vi "Periodic Tasks.vi"(8 "error in":errorcluster) -> ()   [LabVIEW 2018]
doc: "This VI runs in parallel to other tasks. It can contain as many user-defined periodic loops as you need. These can carry out PID or other sorts of timed response."
uses:
  PWF_Venom_LabVIEW/Public/TypeDefs/PwF_Venom_PIDParams.ctl
  DriveVenomDevRefs.ctl
  <vilib>/Rock Robotics/WPI/MotorControl/WPI_MotorControlDeviceRef.ctl
  <vilib>/Rock Robotics/WPI/MotorControl/WPI_MotorControlType.ctl
  <vilib>/Rock Robotics/SystemInterfaces/DIO/FPGA_DIOPWMChannel.ctl
  <vilib>/Rock Robotics/WPI/PWM/WPI_PWMDeadband.ctl
  <vilib>/Rock Robotics/SystemInterfaces/DIO/FPGA_DIOChannel.ctl
  DriveState.ctl
  PWF_Venom_LabVIEW/Public/TypeDefs/PwF_Venom_ControlMode.ctl
  88a8256b-dd6c-4d38-b021-9946be483166.vi
  72a4271e-8a2f-4e63-bef0-ab0047b3c302.vi
  4419bb08-cace-4eec-81e3-431b0f19f77f.vi
  43bb15c8-37b4-49b3-9761-3a694f89d06e.vi
  681b6e5e-4677-4682-a16d-7f94549bf0f7.vi
  f8245736-c666-4745-b76e-80ca56998d75.vi
  eff852b5-78a3-4797-aee6-6215f14f6dac.vi
  <vilib>/Array/Sort 2D Array - Pop Stack.vi
  <vilib>/Array/Sort 2D Array - Push Stack.vi
  <vilib>/Rock Robotics/WPI/Utilities/WPI_GetSetVariantRefNum.vi
  <vilib>/Rock Robotics/Network Tables/NT Read Numeric Array.vi
  <vilib>/Rock Robotics/WPI/ThirdParty/Phoenix-LabVIEW/Pigeon IMU/CTRE_PigeonIMU_GetFusedHeading.vi
  PWF_Venom_LabVIEW/PwF_Venom.lvlib
panel:
  in  "Set Angle":dbl(slide) scale=-180.0..180.0
  out "Degrees Off":dbl
  out "Center":dbl
  out "Height":dbl
  in  "Offset":dbl=182.0
  out "Waveform Chart":dbl(graph)=-0.0
  in  "PID Params":T1={"kP"=0.5, "kI"=0.0, "kD"=0.0, "kF"=0.184, "b"=0.0}
  in  "Track Width":dbl=2.3125
  in  "Tuning":dbl=10.0
  in  "Min Turn Radius":dbl=1.0
  in  "Max Wheel Velocity":dbl=4.0
  out "Avg Left Encoder (ft/s)":dbl
  out "Left Encoder (ft/s)":dbl
  in  "MinPower":dbl=0.063 format="%#_13g"
  out "dTime":u32=31
  out "Speed":dbl
  out "Position":dbl=-0.008333333333333333
  out "RightEncoderInches":dbl=0.005423177083333334
  out "LeftEncoderInches":dbl=0.037962239583333335
  out "RightEncoderRaw":dbl=0.25
  out "LeftEncoderRaw":dbl=1.75
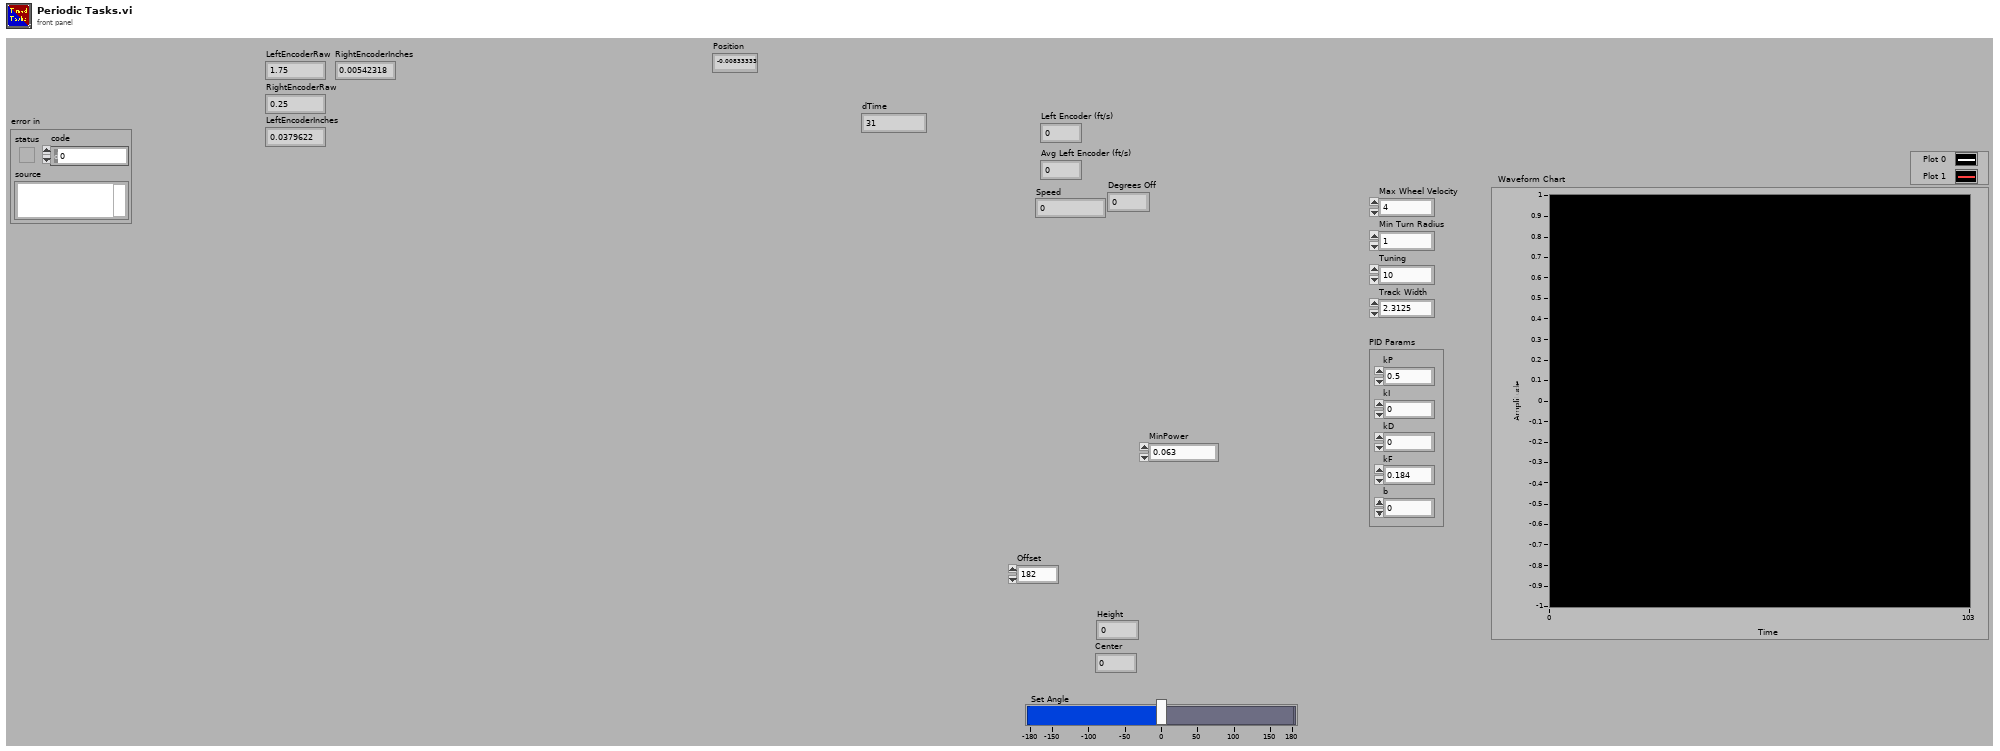
[diagram p1: front panel]
types:
  T1 = typedef "PwF_Venom.lvlib/PwF_Venom_PIDParams.ctl" = cluster{"kP":dbl, "kI":dbl, "kD":dbl, "kF":dbl, "b":dbl}
  T2 = cluster{"millisecond timer value":u32, "Distance":dbl}
  T3 = typedef "DriveVenomDevRefs.ctl" = cluster{"FrontLeft":T4, "FrontRight":T4}
  T4 = typedef "WPI_MotorControlDeviceRef.ctl" = cluster{"DeviceStatus":errorcluster, "Type":T5, "PWM":cluster{"PWM Channel":T6, "DeadBand":T7}, "CAN":cluster{"Device Number":u8, "SetOutput VI Ref":variant, "GetOutput VI Ref":variant, "Enable VI Ref":variant, "Disable VI Ref":variant, "Data":variant}, "Invert":bool, "DIO PWM":cluster{"PWM \"Enable\" Channel":T6, "DIOChannel":T8, "PWM Rate":dbl}}
  T5 = typedef "WPI_MotorControlType.ctl" = enum16{"PWM", "CAN", "DIO PWM"}
  T6 = typedef "FPGA_DIOPWMChannel.ctl" = enum8{"PWM 0", "PWM 1", "PWM 2", "PWM 3", "PWM 4", "PWM 5", "PWM 6", "PWM 7", "PWM 8", "PWM 9", "PWM MXP 0", "PWM MXP 1", "PWM MXP 2", "PWM MXP 3", "PWM MXP 4", "PWM MXP 5", "PWM MXP 6", "PWM MXP 7", "PWM MXP 8", "PWM MXP 9", "Invalid"}
  T7 = typedef "WPI_PWMDeadband.ctl" = cluster{"Name":string, "maxPositivePwm":i32, "minPositivePwm":i32, "centerPwm":i32, "maxNegativePwm":i32, "minNegativePwm":i32, "angularRange":u16}
  T8 = typedef "FPGA_DIOChannel.ctl" = enum8{"DIO 0", "DIO 1", "DIO 2", "DIO 3", "DIO 4", "DIO 5", "DIO 6", "DIO 7", "DIO 8", "DIO 9", "DIO MXP 0", "DIO MXP 1", "DIO MXP 2", "DIO MXP 3", "DIO MXP 4", "DIO MXP 5", "DIO MXP 6", "DIO MXP 7", "DIO MXP 8", "DIO MXP 9", "DIO MXP 10", "DIO MXP 11", "DIO MXP 12", "DIO MXP 13", "DIO MXP 14", "DIO MXP 15", "SPI Port CS1", "SPI Port CS2", "SPI Port CS3", "SPI Port MISO", "SPI Port MOSI", "Invalid"}
  T9 = typedef "WPI_I2CDevRef.ctl" = cluster{"DevStatus":errorcluster, "Device Address":u8, "Handle":i32, "I2C Bus":T10}
  T10 = typedef "i2c_bus.ctl" = enum16{"I2C On-Board", "I2C MXP", "Invalid"}
  T11 = typedef "CTRE_PigeonIMU_DeviceRef.ctl" = cluster{"DeviceStatus":errorcluster, "Device Number":u8, "Type":T12, "Device ID":u32, "Handle":u64, "UsageFrame":u32, "Library Path":path}
  T12 = typedef "CTRE_PigeonIMU_ConnectionType.ctl" = u32
  T13 = typedef "WPI_EncoderDevRef.ctl" = cluster{"DevStatus":errorcluster, "EncoderIndex":T14, "CounterIndex":T15, "DistancePerCount":dbl, "Decoding Type":T16}
  T14 = typedef "FPGA_EncoderIdx.ctl" = enum8{"Enc 0", "Enc 1", "Enc 2", "Enc 3", "Enc 4", "Enc 5", "Enc 6", "Enc 7", "Invalid"}
  T15 = typedef "FPGA_CounterCtrSystemIndex.ctl" = enum8{"Ctr 0", "Ctr 1", "Ctr 2", "Ctr 3", "Ctr 4", "Ctr 5", "Ctr 6", "Ctr 7", "Invalid"}
  T16 = typedef "WPI_EncoderType.ctl" = enum16{"1x", "2x", "4x"}
  T17 = typedef "WPI_JoystickDevRef.ctl" = cluster{"Device":T18}
  T18 = typedef "WPI_JoystickDeviceEnum.ctl" = enum16{"USB 0", "USB 1", "USB 2", "USB 3", "USB 4", "USB 5"}
  T19 = cluster{"millisecond timer value":u32, "Distance":dbl}[]
  T20 = enum16{"[0, 360]", "[-180, 180]", "[0, 2PI]", "[-PI, PI]"}
  T21 = cluster{"Heading":dbl, "Valid?":bool, "Fusing?":bool}
  T22 = typedef "DriveState.ctl" = enum16{"Manual", "Velocity", "Test Static Friction", "Do Nothing"}
  T23 = typedef "PwF_Venom.lvlib/PwF_Venom_ControlMode.ctl" = u8
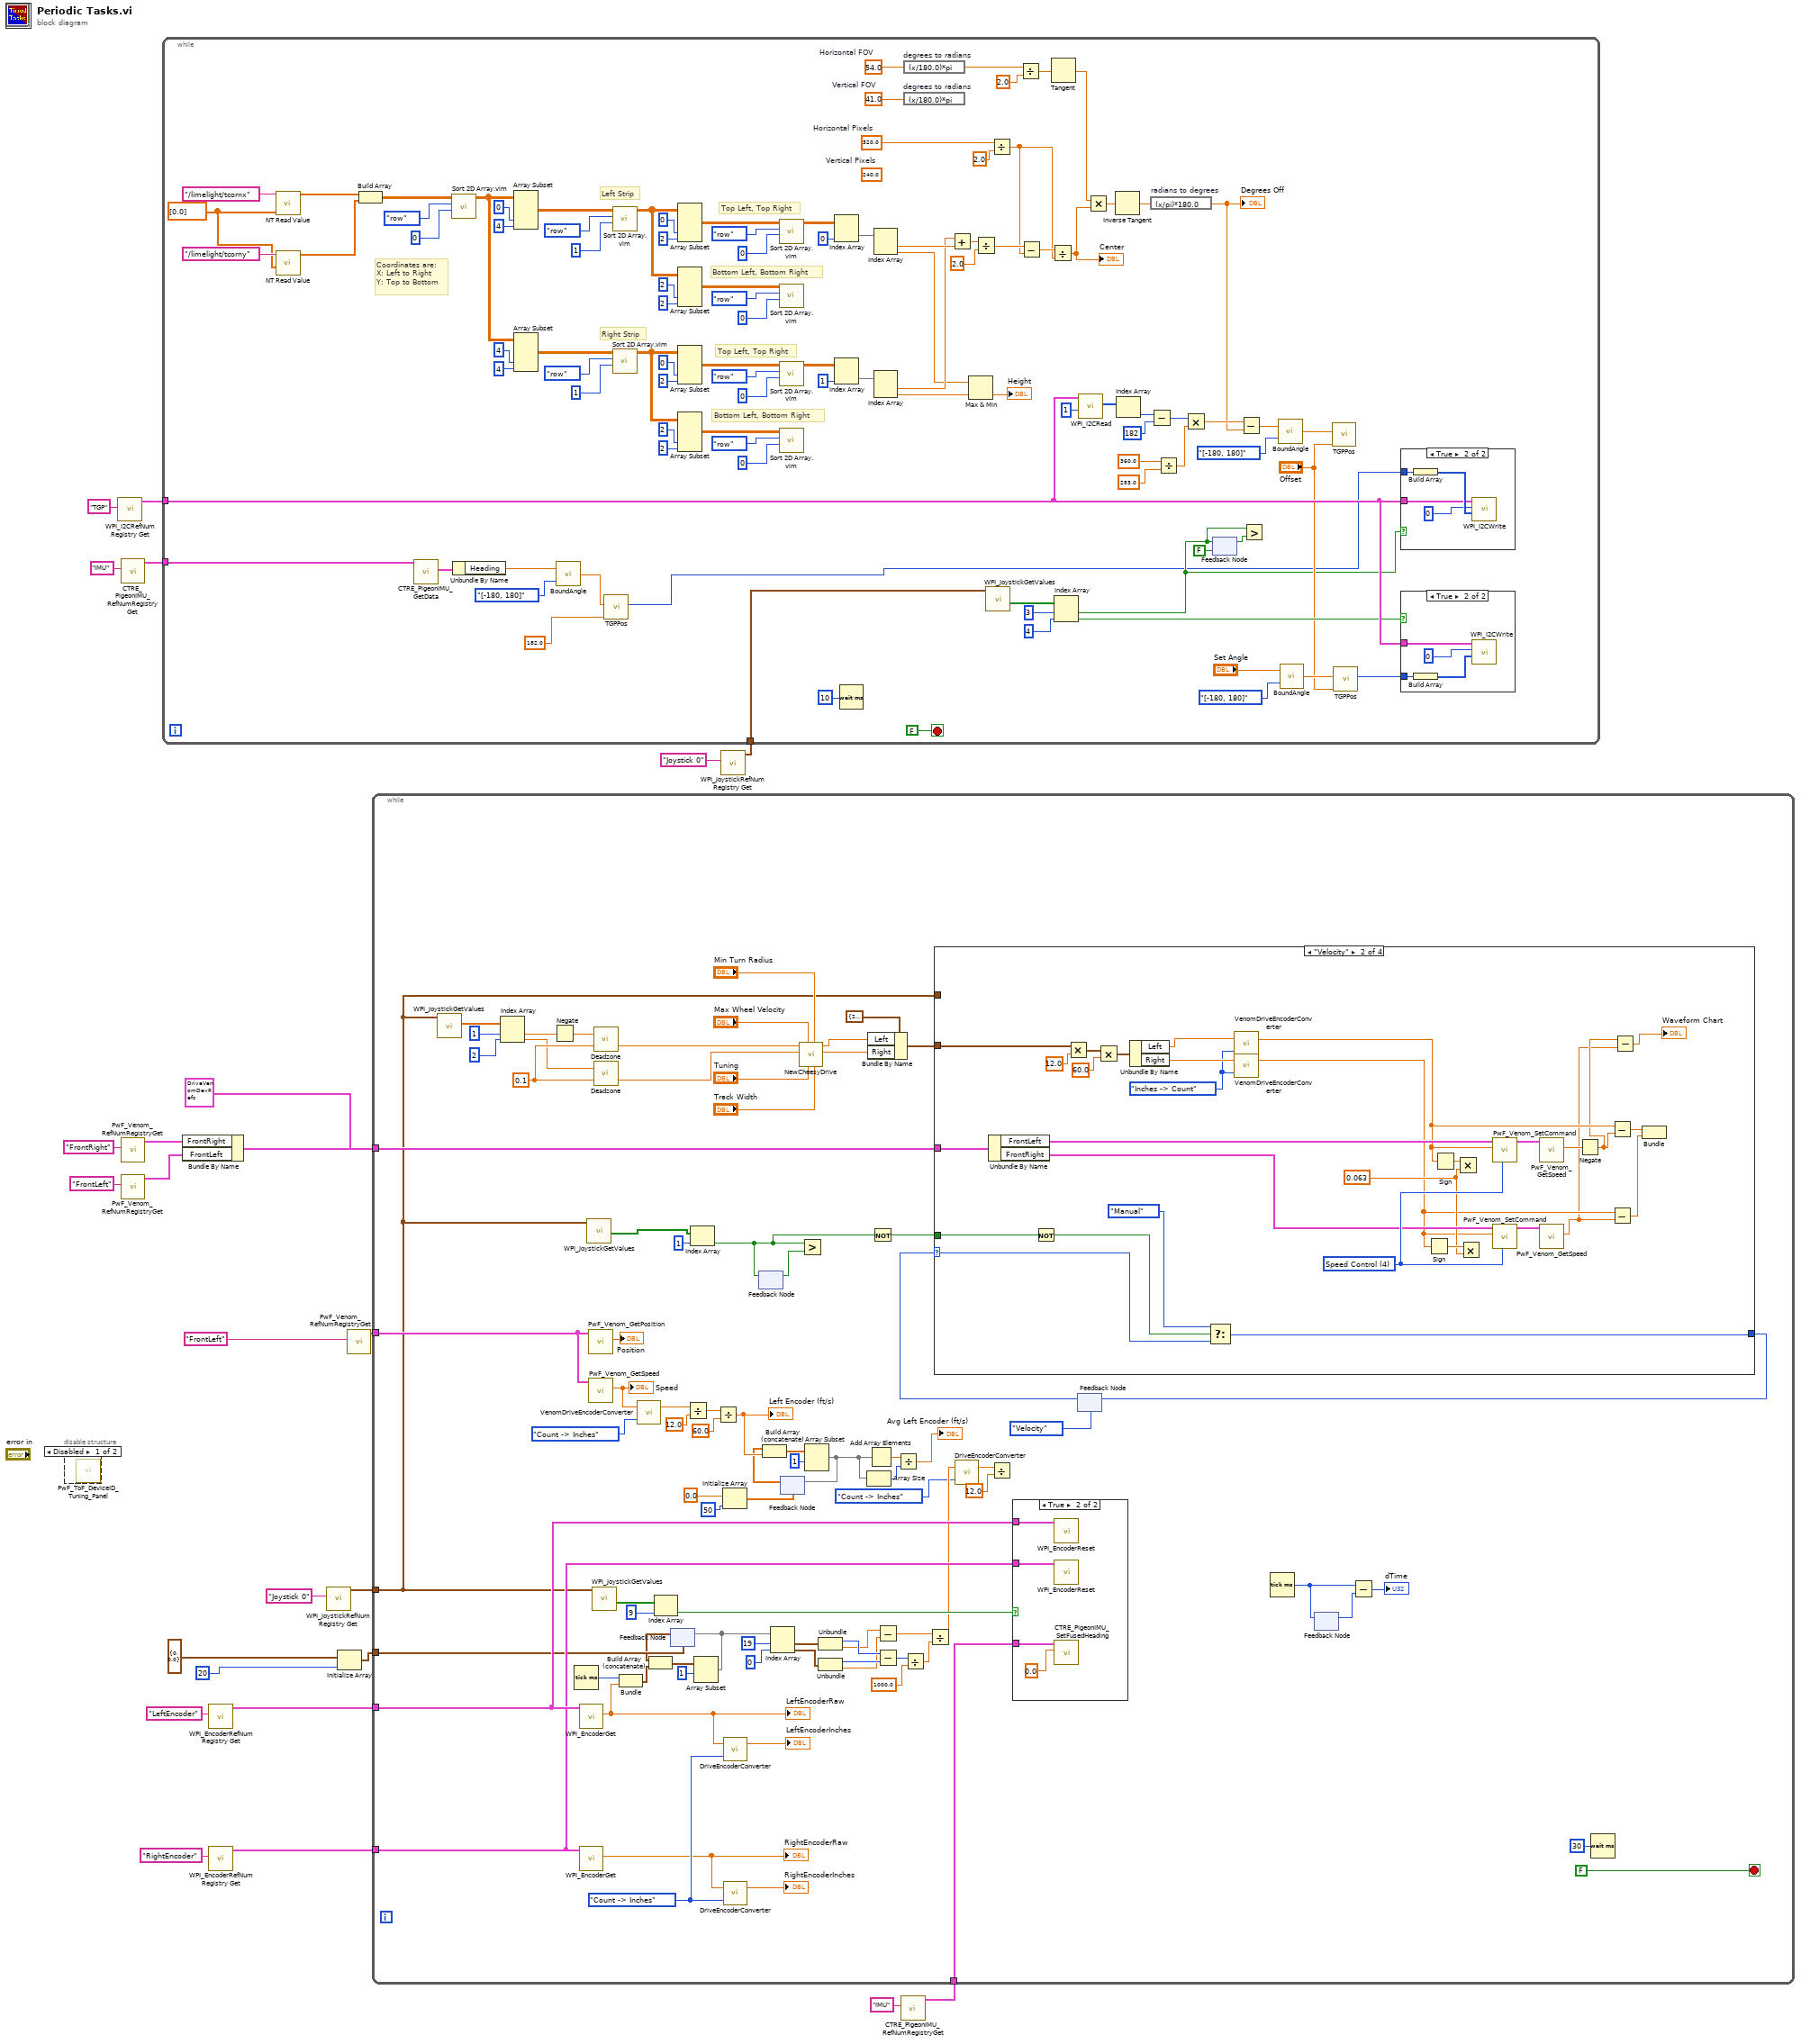
[diagram p0: block diagram]
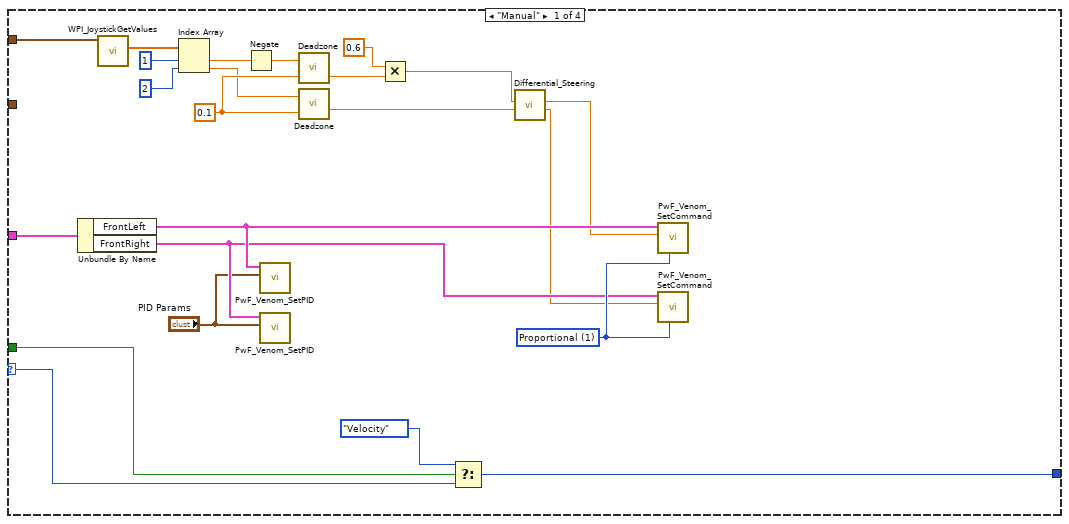
[diagram p6: hidden frame]
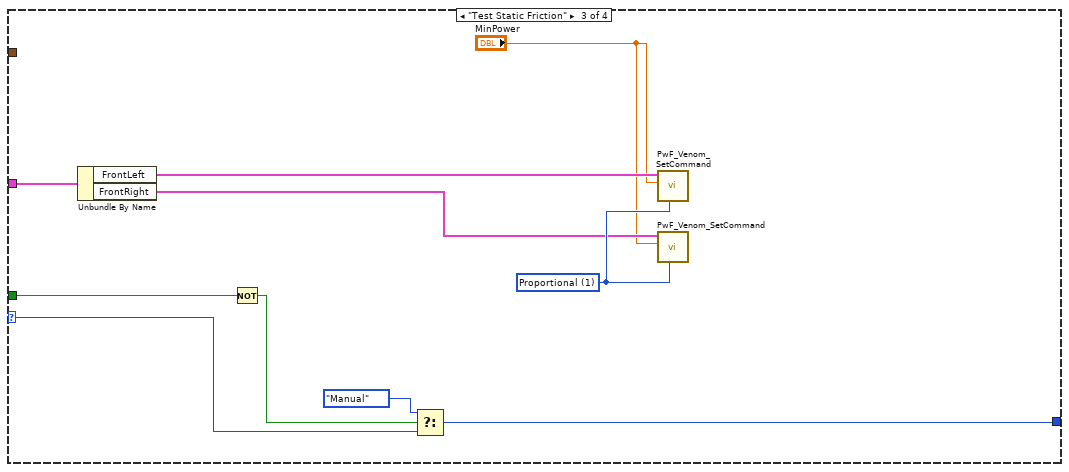
[diagram p7: hidden frame]
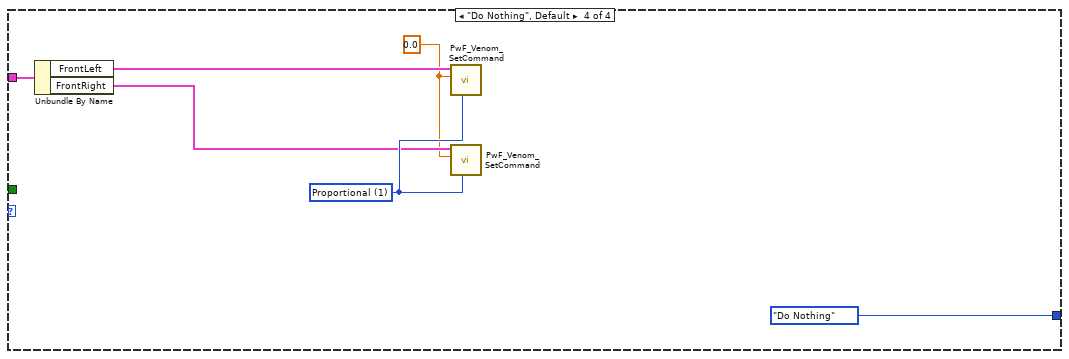
[diagram p8: hidden frame]
diagram:
  n1 = disable-structure shown="Disabled" {
    frame Disabled {
      n2 = call "PwF_ToF_DeviceID_Tuning_Panel.vi"() -> ()  [unwired: 12 in]
    }
    frame Enabled {
    }
  }
  n3 = call <vilib>:"WPI_I2CRefNum Registry Get.vi"("refnum name"="TGP") -> ("I2CDevRef"=w4:T9)  [unwired: 9 in, 1 out]
  n4 = call <vilib>:"CTRE_PigeonIMU_RefNumRegistryGet.vi"("refnum name"="IMU") -> ("PigeonIMUDevRef"=w3:T11)  [unwired: 9 in, 1 out]
  n5 = call "PwF_Venom_RefNumRegistryGet.vi"("refnum name"="FrontRight") -> ("PwFVenomDevRefOut"=w12:T4)  [unwired: 9 in, 1 out]
  n6 = call "PwF_Venom_RefNumRegistryGet.vi"("refnum name"="FrontLeft") -> ("PwFVenomDevRefOut"=w11:T4)  [unwired: 9 in, 1 out]
  n7 = Bundle By Name(cluster=T3 {"FrontLeft"={"DeviceStatus"={"status"=FALSE, "code"=0, "source"=""}, "Type"=enum."PWM", "PWM"={"PWM Channel"=enum."Invalid", "DeadBand"={"Name"="", "maxPositivePwm"=0, "minPositivePwm"=0, "centerPwm"=0, "maxNegativePwm"=0, "minNegativePwm"=0, "angularRange"=0}}, "CAN"={"Device Number"=0, "SetOutput VI Ref"=variant(refnum<vi> refnum), "GetOutput VI Ref"=variant(refnum<vi> refnum), "Enable VI Ref"=variant(refnum<vi> refnum), "Disable VI Ref"=variant(refnum<vi> refnum), "Data"=variant}, "Invert"=FALSE, "DIO PWM"={"PWM \"Enable\" Channel"=enum."Invalid", "DIOChannel"=enum."Invalid", "PWM Rate"=0.0}}, "FrontRight"={"DeviceStatus"={"status"=FALSE, "code"=0, "source"=""}, "Type"=enum."PWM", "PWM"={"PWM Channel"=enum."Invalid", "DeadBand"={"Name"="", "maxPositivePwm"=0, "minPositivePwm"=0, "centerPwm"=0, "maxNegativePwm"=0, "minNegativePwm"=0, "angularRange"=0}}, "CAN"={"Device Number"=0, "SetOutput VI Ref"=variant(refnum<vi> refnum), "GetOutput VI Ref"=variant(refnum<vi> refnum), "Enable VI Ref"=variant(refnum<vi> refnum), "Disable VI Ref"=variant(refnum<vi> refnum), "Data"=variant}, "Invert"=FALSE, "DIO PWM"={"PWM \"Enable\" Channel"=enum."Invalid", "DIOChannel"=enum."Invalid", "PWM Rate"=0.0}}} ("DriveVenomDevRefs"), "FrontRight"=w12, "FrontLeft"=w11) -> (w10:T3)
  n8 = call <vilib>:"WPI_EncoderRefNum Registry Get.vi"("refnum name"="LeftEncoder") -> ("EncoderDevRef"=w24:T13)  [unwired: 9 in, 1 out]
  n9 = call <vilib>:"WPI_EncoderRefNum Registry Get.vi"("refnum name"="RightEncoder") -> ("EncoderDevRef"=w23:T13)  [unwired: 9 in, 1 out]
  n10 = call <vilib>:"WPI_JoystickRefNum Registry Get.vi"("refnum name"="Joystick 0") -> ("JoystickDevRef"=w18:T17)  [unwired: 9 in, 1 out]
  n11 = Initialize Array(T2 {"millisecond timer value"=0, "Distance"=0.0}, 20 ("dimension size")) -> (w7:T19)
  n12 = call "PwF_Venom_RefNumRegistryGet.vi"("refnum name"="FrontLeft") -> ("PwFVenomDevRefOut"=w17:T4)  [unwired: 9 in, 1 out]
  n13 = call <vilib>:"WPI_JoystickRefNum Registry Get.vi"("refnum name"="Joystick 0") -> ("JoystickDevRef"=w1:T17)  [unwired: 9 in, 1 out]
  n14 = while {
    tunnel: w4 -> [w46]
    tunnel: w3 -> [w123]
    tunnel: w1 -> [w35]
    stop <- FALSE stop-if-true
    (unwired) 240.0  # Vertical Pixels
    w58 = 320.0  # Horizontal Pixels
    w67 = 41.0  # Vertical FOV
    w70 = 54.0  # Horizontal FOV
    w118 = dbl[] [0.0] ("Default Value")
    # "Coordinates are:\nX: Left to Right\nY: Top to Bottom"
    # "Top Left, Top Right"
    # "Bottom Left, Bottom Right"
    # "Top Left, Top Right"
    # "Bottom Left, Bottom Right"
    # "Right Strip"
    # "Left Strip"
    n15 = call-poly <vilib>:"NT Read Value.vi"("Default Value"=w118, "Name"="/limelight/tcornx") -> ("Numeric Array"=w120:dbl[])  [unwired: 8 in, 1 out]
    n16 = call-poly <vilib>:"NT Read Value.vi"("Default Value"=w118, "Name"="/limelight/tcorny") -> ("Numeric Array"=w119:dbl[])  [unwired: 8 in, 1 out]
    n17 = Build Array(w120, w119) -> (w115:dbl[][])
    n18 = call-poly <vilib>:"CTRE_PigeonIMU_GetData.vi"("PigeonIMUDevRef"=w123) -> ("Fused Heading"=w125:T21)  [unwired: 8 in, 2 out]
    n19 = call "Sort 2D Array.vim"("index"=0, "dimension to index (column)"=enum16{"column", "row"}."row", "2D array"=w115) -> ("sorted 2D array"=w110:dbl[][])  [unwired: 7 in, 1 out]
    n20 = Unbundle By Name(w125) -> ("Heading"=w126:dbl)
    n21 = Array Subset(array=w110, index (col)=0 ("index"), length (col)=4 ("index")) -> (w107:dbl[][])  [unwired: 2 in]
    n22 = Array Subset(array=w110, index (col)=4 ("index"), length (col)=4 ("index")) -> (w104:dbl[][])  [unwired: 2 in]
    n23 = call <userlib>:"BoundAngle.vi"("Type"=T20."[-180, 180]", "Angle"=w126) -> ("Bound Angle"=w28:dbl)
    n24 = call "TGPPos.vi"("Offset"=182.0 ("Offset 2"), "Angle (-179 - 180)"=w28) -> ("TGP Pos"=w27:u8)  [unwired: 9 in]
    n25 = call "Sort 2D Array.vim"("index"=1, "dimension to index (column)"=enum16{"column", "row"}."row", "2D array"=w107) -> ("sorted 2D array"=w99:dbl[][])  [unwired: 7 in, 1 out]
    n26 = call "Sort 2D Array.vim"("index"=1, "dimension to index (column)"=enum16{"column", "row"}."row", "2D array"=w104) -> ("sorted 2D array"=w94:dbl[][])  [unwired: 7 in, 1 out]
    n27 = Array Subset(array=w99, index (col)=0 ("index"), length (col)=2 ("index")) -> (w91:dbl[][])  [unwired: 2 in]
    n28 = Array Subset(array=w99, index (col)=2 ("index"), length (col)=2 ("index")) -> (w88:dbl[][])  [unwired: 2 in]
    n29 = Array Subset(array=w94, index (col)=0 ("index"), length (col)=2 ("index")) -> (w83:dbl[][])  [unwired: 2 in]
    n30 = Array Subset(array=w94, index (col)=2 ("index"), length (col)=2 ("index")) -> (w82:dbl[][])  [unwired: 2 in]
    n31 = call "Sort 2D Array.vim"("index"=0, "dimension to index (column)"=enum16{"column", "row"}."row", "2D array"=w91) -> ("sorted 2D array"=w79:dbl[][])  [unwired: 7 in, 1 out]
    n32 = call "Sort 2D Array.vim"("index"=0, "dimension to index (column)"=enum16{"column", "row"}."row", "2D array"=w88) -> ()  [unwired: 7 in, 2 out]
    n33 = call "Sort 2D Array.vim"("index"=0, "dimension to index (column)"=enum16{"column", "row"}."row", "2D array"=w83) -> ("sorted 2D array"=w78:dbl[][])  [unwired: 7 in, 1 out]
    n34 = call "Sort 2D Array.vim"("index"=0, "dimension to index (column)"=enum16{"column", "row"}."row", "2D array"=w82) -> ()  [unwired: 7 in, 2 out]
    n35 = Index Array(array=w79, index (col)=0 ("disabled index (col)")) -> (element=w77:dbl[])  [unwired: 1 in]
    n36 = Index Array(array=w78, index (col)=1 ("disabled index (col)")) -> (element=w76:dbl[])  [unwired: 1 in]
    n37 = Wait (ms)(milliseconds to wait=u32 10) -> ()  [unwired: 1 out]
    n38 = Index Array(array=w77) -> (element #1=w75:dbl, element #2=w73:dbl)  [unwired: 2 in]
    n39 = Index Array(array=w76) -> (element #1=w74:dbl, element #2=w72:dbl)  [unwired: 2 in]
    n40 = expression code="(x/180.0)*pi" "degrees to radians"(w70) -> (w68:dbl)
    n41 = expression code="(x/180.0)*pi" "degrees to radians"(w67) -> ()  [unwired: 1 out]
    n42 = Add(x=w74, y=w75) -> (x+y=w62:dbl)
    n43 = Max & Min(x=w73, y=w72) -> (min(x,y)=→"Height":dbl)  [unwired: 1 out]
    n44 = Divide(x=w62, y=2.0 ("x+y")) -> (x/y=w60:dbl)
    n45 = call <vilib>:"WPI_JoystickGetValues.vi"("JoystickDevRef"=w35) -> ("Buttons"=w40:bool[])  [unwired: 6 in, 4 out]
    n46 = Divide(x=w58, y=2.0) -> (x/y=w55:dbl)
    n47 = Divide(x=w68, y=2.0) -> (x/y=w66:dbl)
    n48 = Subtract(x=w60, y=w55) -> (x-y=w59:dbl)
    n49 = Divide(x=w59, y=w55) -> (x/y=w56:dbl)
    "Center" <- w56
    n50 = Tangent(1:w66) -> (0:w65:dbl)
    n51 = Index Array(array=w40, index #1=3 ("index"), index #2=4 ("index")) -> (element #1=w29:bool, element #2=w36:bool)
    n52 = call <vilib>:"WPI_I2CRead.vi"("I2CBytesToRead"=u8 1, "I2CDevRef"=w46) -> ("Data Out"=w54:u8[])  [unwired: 7 in, 2 out]
    n53 = Multiply(x=w65, y=w56) -> (x*y=w64:dbl)
    n54 = Inverse Tangent(1:w64) -> (0:w63:dbl)
    n55 = Index Array(array=w54) -> (element=w51:u8)  [unwired: 1 in]
    n56 = Subtract(x=w51, y=u8 182) -> (x-y=w32:u8)
    n57 = expression code="(x/pi)*180.0" "radians to degrees"(w63) -> (w33:dbl)
    "Degrees Off" <- w33
    n58 = Divide(x=360.0, y=253.0 ("x")) -> (x/y=w50:dbl)
    n59 = Multiply(x=w32, y=w50) -> (x*y=w34:dbl)
    n60 = feedback-in #1(w29) -> ()
    n61 = feedback #1(FALSE) -> (w38:bool)
    n62 = Subtract(x=w34, y=w33) -> (x-y=w48:dbl)
    n63 = Greater?(x=w29, y=w38) -> ()  [unwired: 1 out]
    n64 = call <userlib>:"BoundAngle.vi"("Type"=T20."[-180, 180]", "Angle"=w48) -> ("Bound Angle"=w47:dbl)
    n65 = call <userlib>:"BoundAngle.vi"("Type"=T20."[-180, 180]", "Angle"="Set Angle") -> ("Bound Angle"=w44:dbl)
    n66 = call "TGPPos.vi"("Offset"="Offset", "Angle (-179 - 180)"=w47) -> ()  [unwired: 9 in, 1 out]
    n67 = call "TGPPos.vi"("Offset"="Offset", "Angle (-179 - 180)"=w44) -> ("TGP Pos"=w42:u8)  [unwired: 9 in]
    n68 = case shown="True" w29 {
      tunnel: w46 -> [_ w135]
      tunnel: w27 -> [_ w134]
      frame False {
      }
      frame True {
        n69 = Build Array(w134) -> (w137:u8[])
        n70 = call <vilib>:"WPI_I2CWrite.vi"("I2CDataToSend"=w137, "I2CRegister"=u8 0, "I2CDevRef"=w135) -> ()  [unwired: 7 in, 2 out]
      }
    }
    n71 = case shown="True" w36 {
      tunnel: w42 -> [_ w131]
      tunnel: w46 -> [_ w130]
      frame False {
      }
      frame True {
        n72 = Build Array(w131) -> (w133:u8[])
        n73 = call <vilib>:"WPI_I2CWrite.vi"("I2CDataToSend"=w133, "I2CRegister"=u8 0, "I2CDevRef"=w130) -> ()  [unwired: 7 in, 2 out]
      }
    }
  }
  n74 = call <vilib>:"CTRE_PigeonIMU_RefNumRegistryGet.vi"("refnum name"="IMU") -> ("PigeonIMUDevRef"=w20:T11)  [unwired: 9 in, 1 out]
  n75 = while {
    tunnel: w24 -> [w220]
    tunnel: w23 -> [w219]
    tunnel: w20 -> [w218]
    tunnel: w18 -> [w187]
    tunnel: w17 -> [w217]
    tunnel: w10 -> [w216]
    tunnel: w7 -> [w209]
    stop <- FALSE stop-if-true
    w186 = enum16{"Count -> Inches", "Inches -> Count"}."Count -> Inches" ("Mode")
    w196 = 0.1 ("Deadzone")
    n76 = call <vilib>:"WPI_JoystickGetValues.vi"("JoystickDevRef"=w187) -> ("Axes"=w197:dbl[])  [unwired: 6 in, 4 out]
    n77 = Index Array(array=w197, index #1=1 ("index"), index #2=2 ("index")) -> (element #1=w198:dbl, element #2=w192:dbl)
    n78 = Negate(x=w198) -> (-x=w193:dbl)
    n79 = Tick Count (ms)() -> (millisecond timer value=w172:u32)
    n80 = call <vilib>:"WPI_EncoderGet.vi"("EncoderDevRef"=w220) -> ("Distance"=w173:dbl)  [unwired: 5 in, 5 out]
    "LeftEncoderRaw" <- w173
    n81 = call <vilib>:"WPI_EncoderGet.vi"("EncoderDevRef"=w219) -> ("Distance"=w181:dbl)  [unwired: 5 in, 5 out]
    "RightEncoderRaw" <- w181
    n82 = call <vilib>:"WPI_JoystickGetValues.vi"("JoystickDevRef"=w187) -> ("Buttons"=w188:bool[])  [unwired: 6 in, 4 out]
    n83 = call "PwF_Venom_GetPosition.vi"("PwFVenomDevRefIn"=w217) -> ("Position"=→"Position":dbl)  [unwired: 8 in, 2 out]
    n84 = call "PwF_Venom_GetSpeed.vi"("PwFVenomDevRefIn"=w217) -> ("Speed"=w142:dbl)  [unwired: 8 in, 2 out]
    "Speed" <- w142
    n85 = call <vilib>:"WPI_JoystickGetValues.vi"("JoystickDevRef"=w187) -> ("Buttons"=w177:bool[])  [unwired: 6 in, 4 out]
    n86 = call <userlib>:"Deadzone.vi"("Deadzone"=w196, "Input Signal"=w193) -> ("Output Signal"=w191:dbl)  [unwired: 1 out]
    n87 = call <userlib>:"Deadzone.vi"("Deadzone"=w196, "Input Signal"=w192) -> ("Output Signal"=w190:dbl)  [unwired: 1 out]
    n88 = Bundle("millisecond timer value"=w172, "Distance"=w173) -> (w171:T2)  [unwired: 1 in]
    n89 = call "VenomDriveEncoderConverter.vi"("Mode"=enum16{"Count -> Inches", "Inches -> Count"}."Count -> Inches", "Input"=w142) -> ("Output"=w141:dbl)  [unwired: 1 in]
    n90 = Index Array(array=w177, index=9) -> (element=w182:bool)
    n91 = feedback #2(w209) -> (w174:T19)
    n92 = Build Array (concatenate)(w174, w171) -> (w176:T19)
    n93 = Divide(x=w141, y=12.0) -> (x/y=w139:dbl)
    n94 = Index Array(array=w188, index=1) -> (element=w210:bool)
    n95 = Array Subset(array=w176, index=1) -> (w170:T19)  [unwired: 1 in]
    n96 = feedback-in #2(w170) -> ()
    n97 = Divide(x=w139, y=60.0) -> (x/y=w208:dbl)
    "Left Encoder (ft/s)" <- w208
    n98 = Initialize Array(0.0 ("y"), 50 ("dimension size")) -> (w148:dbl[])
    n99 = call "DriveEncoderConverter.vi"("Mode"=w186, "Input"=w173) -> ("Output"=→"LeftEncoderInches":dbl)  [unwired: 1 in]
    n100 = call "DriveEncoderConverter.vi"("Mode"=w186, "Input"=w181) -> ("Output"=→"RightEncoderInches":dbl)  [unwired: 1 in]
    n101 = feedback-in #3(w210) -> ()
    n102 = feedback #3() -> (w211:bool)  [unwired: 1 in]
    n103 = Index Array(array=w170, index #1=19 ("index"), index #2=0 ("index")) -> (element #1=w167:T2, element #2=w166:T2)
    n104 = feedback #4(w148) -> (w151:dbl[])
    n105 = Build Array (concatenate)(w151, w208) -> (w153:dbl[])
    n106 = call "NewCheesyDrive.vi"("Track Width"="Track Width", "Min Turn Radius"="Min Turn Radius", "Tuning"="Tuning", "Max Wheel Velocity"="Max Wheel Velocity", "X"=w190, "Y"=w191) -> ("Right Speed"=w204:dbl, "Left Speed"=w203:dbl)  [unwired: 4 in]
    n107 = Greater?(x=w210, y=w211) -> ()  [unwired: 1 out]
    n108 = Array Subset(array=w153, index=1) -> (w147:dbl[])  [unwired: 1 in]
    n109 = feedback-in #4(w147) -> ()
    n110 = Unbundle(w167) -> ("millisecond timer value"=w165:u32, "Distance"=w163:dbl)
    n111 = Unbundle(w166) -> ("millisecond timer value"=w164:u32, "Distance"=w162:dbl)
    n112 = Array Size(array=w147) -> (size(s)=w145:i32)
    n113 = Bundle By Name(cluster=cluster{"Left":dbl, "Right":dbl} {"Left"=2.0, "Right"=2.0} ("input cluster"), "Left"=w203, "Right"=w204) -> (w205:cluster{"Left":dbl, "Right":dbl})
    n114 = Add Array Elements(numeric array=w147) -> (sum=w146:dbl)
    n115 = Not(x=w210) -> (.not. x?=w189:bool)
    n116 = Subtract(x=w163, y=w162) -> (x-y=w161:dbl)
    n117 = Subtract(x=w165, y=w164) -> (x-y=w156:u32)
    n118 = Divide(x=w146, y=w145) -> (x/y=→"Avg Left Encoder (ft/s)":dbl)
    n119 = Divide(x=w156, y=1000.0) -> (x/y=w155:dbl)
    n120 = Divide(x=w161, y=w155) -> (x/y=w160:dbl)
    n121 = call "DriveEncoderConverter.vi"("Mode"=enum16{"Count -> Inches", "Inches -> Count"}."Count -> Inches", "Input"=w160) -> ("Output"=w158:dbl)  [unwired: 1 in]
    n122 = Divide(x=w158, y=12.0) -> ()  [unwired: 1 out]
    n123 = case shown="True" w182 {
      tunnel: w220 -> [_ w226]
      tunnel: w219 -> [_ w225]
      tunnel: w218 -> [_ w224]
      frame False {
      }
      frame True {
        n124 = call <vilib>:"WPI_EncoderReset.vi"("EncoderDevRef"=w226) -> ()  [unwired: 9 in, 2 out]
        n125 = call <vilib>:"WPI_EncoderReset.vi"("EncoderDevRef"=w225) -> ()  [unwired: 9 in, 2 out]
        n126 = call <vilib>:"CTRE_PigeonIMU_SetFusedHeading.vi"("Value"=0.0, "PigeonIMUDevRef 2"=w224) -> ()  [unwired: 8 in, 2 out]
      }
    }
    n127 = feedback #5(DriveState."Velocity") -> (w214:T22)
    n128 = case shown="\"Velocity\"" w214 {
      selector: w214 -> [w235 w274 w283 _]
      tunnel: w187 -> [w243 _ _ _]
      tunnel: w216 -> [w242 w278 w288 w294]
      tunnel: w205 -> [_ w265 _ _]
      tunnel: [w237 w275 w284 DriveState."Do Nothing"] -> w213
      tunnel: w189 -> [w236 w273 w282 _]
      frame "Manual" {
        w247 = 0.1 ("Deadzone")
        w246 = T23 1 items=["Disabled"=0, "Proportional"=1, "Current Control"=3, "Speed Control"=4, "Position Control"=5, "Motion Profile"=6, "Follow The Leader"=7, "Voltage Control"=8] ("PwF Venom Control Mode")
        n129 = Unbundle By Name(w242) -> ("FrontLeft"=w233:T4, "FrontRight"=w232:T4)
        n130 = call <vilib>:"WPI_JoystickGetValues.vi"("JoystickDevRef"=w243) -> ("Axes"=w248:dbl[])  [unwired: 6 in, 4 out]
        n131 = Index Array(array=w248, index #1=1 ("index"), index #2=2 ("index")) -> (element #1=w249:dbl, element #2=w239:dbl)
        n132 = Negate(x=w249) -> (-x=w241:dbl)
        n133 = call "PwF_Venom_SetPID.vi"("PID Params"="PID Params", "PwFVenomDevRefIn"=w233) -> ()  [unwired: 8 in, 2 out]
        n134 = call "PwF_Venom_SetPID.vi"("PID Params"="PID Params", "PwFVenomDevRefIn"=w232) -> ()  [unwired: 8 in, 2 out]
        n135 = call <userlib>:"Deadzone.vi"("Deadzone"=w247, "Input Signal"=w241) -> ("Output Signal"=w240:dbl)  [unwired: 1 out]
        n136 = call <userlib>:"Deadzone.vi"("Deadzone"=w247, "Input Signal"=w239) -> ("Output Signal"=w228:dbl)  [unwired: 1 out]
        n137 = Multiply(x=0.6, y=w240) -> (x*y=w227:dbl)
        n138 = Select(t=DriveState."Velocity", s=w236, f=w235) -> (s? t:f=w237:T22)
        n139 = call <userlib>:"Differential_Steering.vi"("Steer"=w228, "Base"=w227) -> ("Right"=w229:dbl, "Left"=w230:dbl)  [unwired: 4 in]
        n140 = call "PwF_Venom_SetCommand.vi"("PwF Venom Control Mode"=w246, "command"=w230, "PwFVenomDevRefIn"=w233) -> ()  [unwired: 7 in, 2 out]
        n141 = call "PwF_Venom_SetCommand.vi"("PwF Venom Control Mode"=w246, "command"=w229, "PwFVenomDevRefIn"=w232) -> ()  [unwired: 7 in, 2 out]
      }
      frame "Velocity" {
        w261 = enum16{"Count -> Inches", "Inches -> Count"}."Inches -> Count" ("Mode")
        w269 = 0.063
        w279 = T23 4 items=["Disabled"=0, "Proportional"=1, "Current Control"=3, "Speed Control"=4, "Position Control"=5, "Motion Profile"=6, "Follow The Leader"=7, "Voltage Control"=8] ("PwF Venom Control Mode")
        n142 = Unbundle By Name(w278) -> ("FrontLeft"=w277:T4, "FrontRight"=w276:T4)
        n143 = Not(x=w273) -> (.not. x?=w260:bool)
        n144 = Multiply(x=w265, y=12.0) -> (x*y=w267:cluster{"Left":dbl, "Right":dbl})
        n145 = Multiply(x=w267, y=60.0) -> (x*y=w264:cluster{"Left":dbl, "Right":dbl})
        n146 = Unbundle By Name(w264) -> ("Left"=w262:dbl, "Right"=w263:dbl)
        n147 = Select(t=DriveState."Manual", s=w260, f=w274) -> (s? t:f=w275:T22)
        n148 = call "VenomDriveEncoderConverter.vi"("Mode"=w261, "Input"=w262) -> ("Output"=w254:dbl)  [unwired: 1 in]
        n149 = call "VenomDriveEncoderConverter.vi"("Mode"=w261, "Input"=w263) -> ("Output"=w253:dbl)  [unwired: 1 in]
        n150 = Sign(1:w253) -> (0:w270:dbl)
        n151 = Sign(1:w254) -> (0:w271:dbl)
        n152 = Multiply(x=w271, y=w269) -> ()  [unwired: 1 out]
        n153 = Multiply(x=w270, y=w269) -> ()  [unwired: 1 out]
        n154 = call "PwF_Venom_SetCommand.vi"("PwF Venom Control Mode"=w279, "command"=w254, "PwFVenomDevRefIn"=w277) -> ("PwFVenomDevRefOut"=w255:T4)  [unwired: 7 in, 1 out]
        n155 = call "PwF_Venom_SetCommand.vi"("PwF Venom Control Mode"=w279, "command"=w253, "PwFVenomDevRefIn"=w276) -> ("PwFVenomDevRefOut"=w256:T4)  [unwired: 7 in, 1 out]
        n156 = call "PwF_Venom_GetSpeed.vi"("PwFVenomDevRefIn"=w255) -> ("Speed"=w259:dbl)  [unwired: 8 in, 2 out]
        n157 = call "PwF_Venom_GetSpeed.vi"("PwFVenomDevRefIn"=w256) -> ("Speed"=w251:dbl)  [unwired: 8 in, 2 out]
        n158 = Negate(x=w259) -> (-x=w252:dbl)
        n159 = Subtract(x=w254, y=w252) -> (x-y=w258:dbl)
        n160 = Subtract(x=w253, y=w251) -> (x-y=w257:dbl)
        n161 = Subtract(x=w252, y=w251) -> (x-y=→"Waveform Chart":dbl)
        n162 = Bundle(w258, w257) -> ()  [unwired: 1 in, 1 out]
      }
      frame "Test Static Friction" {
        w289 = T23 1 items=["Disabled"=0, "Proportional"=1, "Current Control"=3, "Speed Control"=4, "Position Control"=5, "Motion Profile"=6, "Follow The Leader"=7, "Voltage Control"=8] ("PwF Venom Control Mode")
        n163 = Unbundle By Name(w288) -> ("FrontLeft"=w287:T4, "FrontRight"=w286:T4)
        n164 = Not(x=w282) -> (.not. x?=w281:bool)
        n165 = Select(t=DriveState."Manual", s=w281, f=w283) -> (s? t:f=w284:T22)
        n166 = call "PwF_Venom_SetCommand.vi"("PwF Venom Control Mode"=w289, "command"="MinPower", "PwFVenomDevRefIn"=w287) -> ()  [unwired: 7 in, 2 out]
        n167 = call "PwF_Venom_SetCommand.vi"("PwF Venom Control Mode"=w289, "command"="MinPower", "PwFVenomDevRefIn"=w286) -> ()  [unwired: 7 in, 2 out]
      }
      frame "Do Nothing", Default {
        w291 = 0.0 ("command")
        w295 = T23 1 items=["Disabled"=0, "Proportional"=1, "Current Control"=3, "Speed Control"=4, "Position Control"=5, "Motion Profile"=6, "Follow The Leader"=7, "Voltage Control"=8] ("PwF Venom Control Mode")
        n168 = Unbundle By Name(w294) -> ("FrontLeft"=w293:T4, "FrontRight"=w292:T4)
        n169 = call "PwF_Venom_SetCommand.vi"("PwF Venom Control Mode"=w295, "command"=w291, "PwFVenomDevRefIn"=w293) -> ()  [unwired: 7 in, 2 out]
        n170 = call "PwF_Venom_SetCommand.vi"("PwF Venom Control Mode"=w295, "command"=w291, "PwFVenomDevRefIn"=w292) -> ()  [unwired: 7 in, 2 out]
      }
    }
    n171 = feedback-in #5(w213) -> ()
    n172 = Tick Count (ms)() -> (millisecond timer value=w179:u32)
    n173 = feedback #6() -> (w180:u32)  [unwired: 1 in]
    n174 = feedback-in #6(w179) -> ()
    n175 = Subtract(x=w179, y=w180) -> (x-y=→"dTime":u32)
    n176 = Wait (ms)(milliseconds to wait=u32 30) -> ()  [unwired: 1 out]
  }
